vi "write_fifo_resonance.vi"(5 "enable fly-back reversion?":bool, 7 "fly-back?":bool, 8 "pixel finished?":bool, 10 "maximum bit depth":i8, 11 "integration cluster in":T1) -> (0 "FIFO overflow out":bool, 3 "integration cluster out":T1)   [LabVIEW 2010]
uses:
  integration_cluster.ctl
  <vilib>/rvi/DataTransferAndStorage/Container/XNode/niFpgaContainer.xnode
  <vilib>/rvi/DataTransferAndStorage/Container/Common/niFpgaContainerMethod.ctl
  <vilib>/rvi/DataTransferAndStorage/Container/Common/niFpgaTransferTypeControl.ctl
  <vilib>/rvi/Memory/Memory_Emulation/nirvimemoryEmulationManagerCache_GetValue.vi
  <vilib>/rvi/DataTransferAndStorage/Container/Common/niFpgaContainerGetUniqueNameForEmu.vi
  <vilib>/rvi/Memory/Memory_Emulation/nirvimemoryEmulationManagerCache_InsertValue.vi
  <vilib>/Utility/error.llb/Clear Errors.vi
  <vilib>/rvi/Memory/Memory_Emulation/nirvimemoryEmulationManagerCache_SetValue.vi
  <vilib>/rvi/interface/RandomDataEmulation/nirviRandomDataFPGAFIFO.vi
  <vilib>/rvi/interface/RandomDataEmulation/niFpgaRandomDataHandleErrors.vi
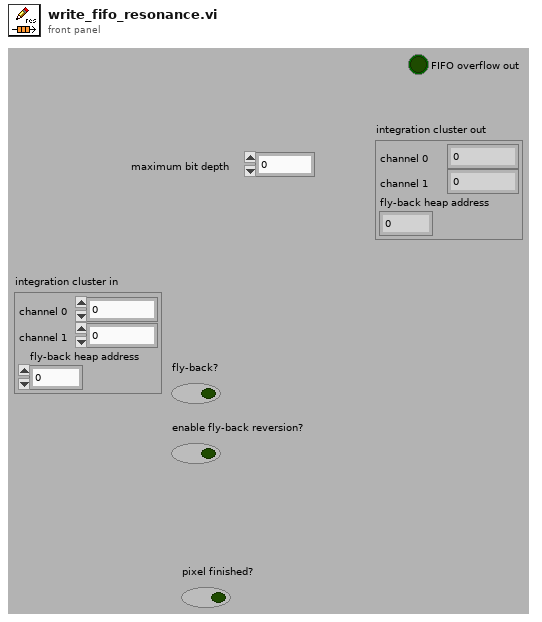
[diagram p1: front panel]
types:
  T1 = typedef "integration_cluster.ctl" = cluster{"channel 0":u32, "channel 1":u32, "fly-back heap address":u32}
  T2 = typedef "niFpgaContainerMethod.ctl" = enum16{"<none>", "write", "read", "clear", "getNumberOfElementsToWrite", "getNumberOfElementsToRead", "enable", "disable", "flushAndDisable", "getStreamState", "readA", "readB", "dramWrite", "dramWriteWithByteEnables", "dramRequestData", "dramRetrieveData"}
  T3 = typedef "niFpgaTransferTypeControl.ctl" = enum16{"Target-Scoped", "Host to Target - DMA", "Target to Host - DMA", "Peer to Peer Reader", "Peer to Peer Writer", "Bidirectional"}
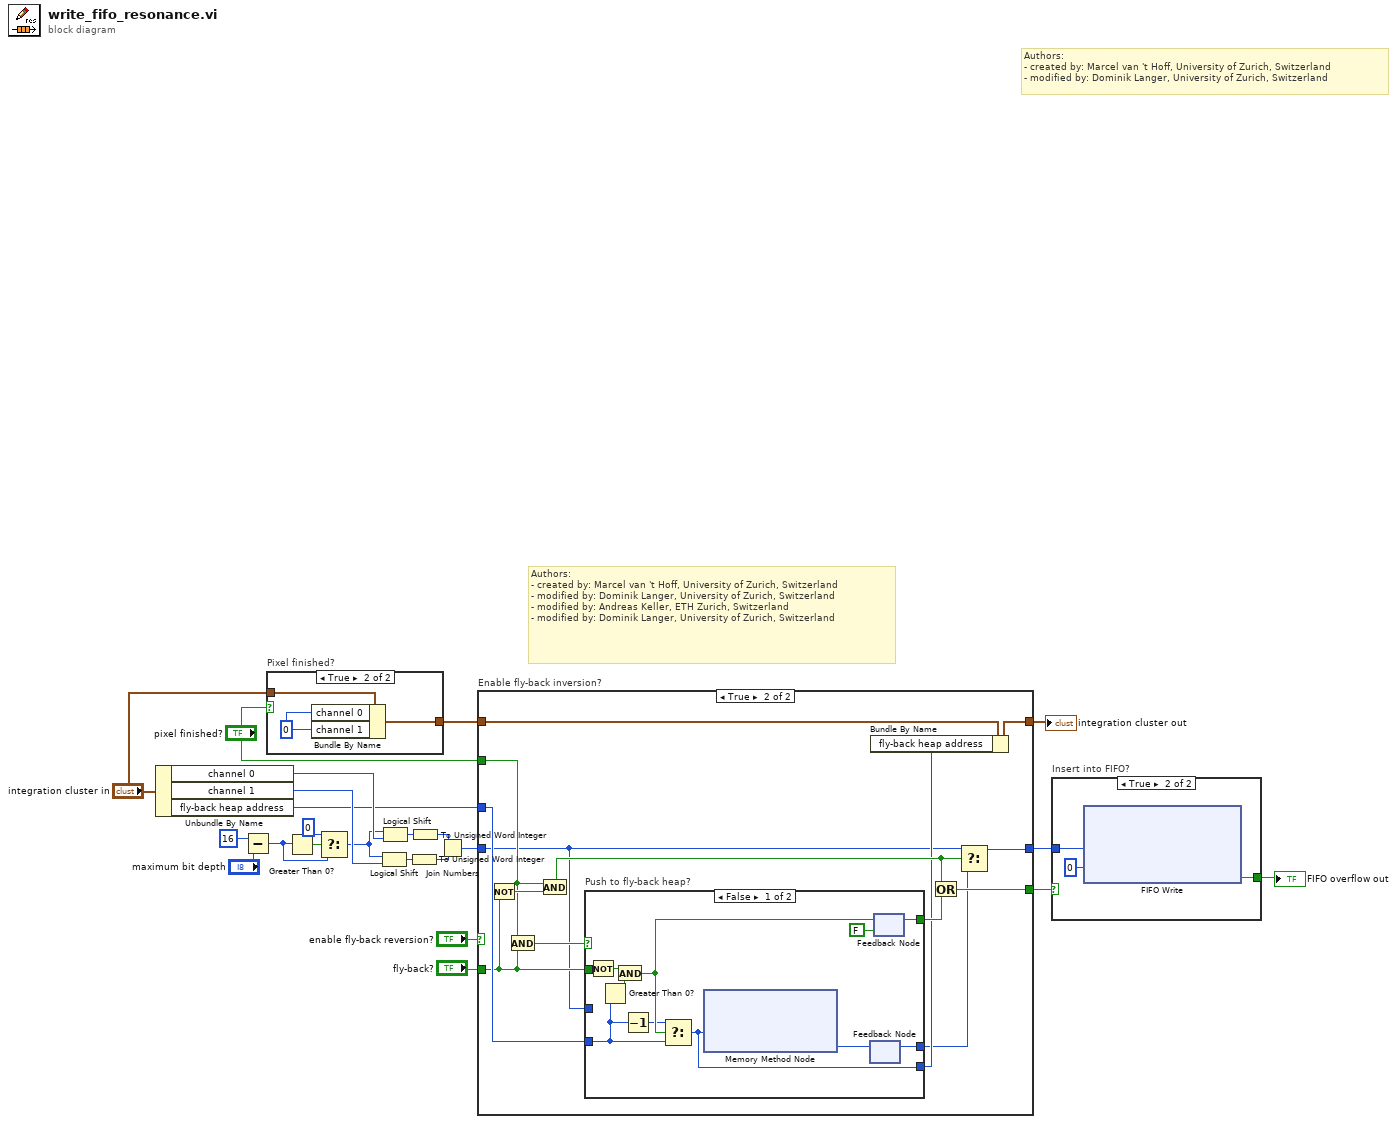
[diagram p0: block diagram]
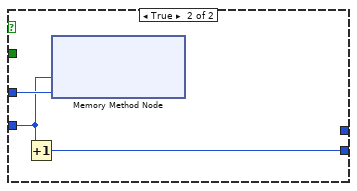
[diagram p4: hidden frame]
diagram:
  # "Authors: \n- created by: Marcel van 't Hoff, University of Zurich, Switzerland\n- modified by: Dominik Langer, University of Zurich, Switzerland\n- modified by: Andreas Keller, ETH Zurich, Switzerland\n- modified by: Dominik Langer, University of Zurich, Switzerland"
  # "Authors: \n- created by: Marcel van 't Hoff, University of Zurich, Switzerland\n- modified by: Dominik Langer, University of Zurich, Switzerland"
  n1 = Unbundle By Name("integration cluster in") -> ("channel 0"=w16:u32, "channel 1"=w17:u32, "fly-back heap address"=w6:u32)
  n2 = Subtract(x=i8 16, y="maximum bit depth") -> (x-y=w19:i8)
  n3 = case "Pixel finished?" shown="True" "pixel finished?" {
    tunnel: "integration cluster in" -> [w24 w26]
    tunnel: [w24 w25] -> w3
    frame False {
    }
    frame True {
      w27 = u32 0 ("channel 1")
      n4 = Bundle By Name(cluster=w26, "channel 0"=w27, "channel 1"=w27) -> (w25:T1)
    }
  }
  n5 = Greater Than 0?(x=w19) -> (x > 0?=w18:bool)
  n6 = Select(t=i8 0 ("f"), s=w18, f=w19) -> (s? t:f=w15:i8)
  n7 = Logical Shift(y=w15, x=w17) -> (x << y=w14:u32)
  n8 = Logical Shift(y=w15, x=w16) -> (x << y=w13:u32)
  n9 = To Unsigned Word Integer(number=w14) -> (unsigned 16bit integer=w11:u16)
  n10 = To Unsigned Word Integer(number=w13) -> (unsigned 16bit integer=w12:u16)
  n11 = Join Numbers(hi=w12, lo=w11) -> ((hi.lo)=w10:u32)
  n12 = case "Enable fly-back inversion?" shown="True" "enable fly-back reversion?" {
    tunnel: w6 -> [_ w44]
    tunnel: w10 -> [w30 w33]
    tunnel: [w30 w42] -> w9
    tunnel: "pixel finished?" -> [w29 w37]
    tunnel: [w29 w32] -> w5
    tunnel: "fly-back?" -> [_ w39]
    tunnel: w3 -> [w28 w36]
    tunnel: [w28 w34] -> w1
    frame False {
    }
    frame True {
      n13 = Not(x=w39) -> (.not. x?=w43:bool)
      n14 = And(x=w37, y=w39) -> (x .and. y?=w41:bool)
      n15 = And(x=w37, y=w43) -> (x .and. y?=w40:bool)
      n16 = case "Push to fly-back heap?" shown="False" w41 {
        tunnel: w33 -> [_ w184]
        tunnel: [w45 w183] -> w35
        tunnel: w44 -> [w47 w182]
        tunnel: w39 -> [w54 _]
        tunnel: [w50 _] -> w31
        tunnel: [w52 _] -> w38
        frame False {
          n17 = Not(x=w54) -> (.not. x?=w53:bool)
          n18 = Greater Than 0?(x=w47) -> (x > 0?=w55:bool)
          n19 = And(x=w53, y=w55) -> (x .and. y?=w48:bool)
          n20 = Decrement(x=w47) -> (x-1=w46:u32)
          n21 = Select(t=w46, s=w48, f=w47) -> (s? t:f=w45:u32)
          n22 = xnode ("Memory Method Node")("Address"=w45) -> ("Data"=w49:u32)  [unwired: 1 in, 1 out]
          n23 = feedback #1() -> (w50:u32)  [unwired: 1 in]
          n24 = feedback-in #1(w49) -> ()
          n25 = feedback #2(FALSE) -> (w52:bool)
          n26 = feedback-in #2(w48) -> ()
        }
        frame True {
          n27 = Increment(x=w182) -> (x+1=w183:u32)
          n28 = xnode ("Memory Method Node")("Address"=w182, "Data"=w184) -> ()  [unwired: 1 in, 1 out]
        }
      }
      n29 = Bundle By Name(cluster=w36, "fly-back heap address"=w35) -> (w34:T1)
      n30 = Or(x=w40, y=w38) -> (x .or. y?=w32:bool)
      n31 = Select(t=w33, s=w40, f=w31) -> (s? t:f=w42:u32)
    }
  }
  "integration cluster out" <- w1
  n32 = case "Insert into FIFO?" shown="True" w5 {
    tunnel: [_ w312] -> w22
    tunnel: w9 -> [_ w310]
    frame False {
    }
    frame True {
      n33 = xnode ("FIFO Write")("Element"=w310, "Timeout"=0) -> ("Timed Out?"=w312:bool)  [unwired: 1 in, 1 out]
    }
  }
  "FIFO overflow out" <- w22
